vi "SMTP Email [VRFY].vi"(4 "error in (no error)":errorcluster, 6 "user":string, 7 "smtp session":T1) -> (0 "error out":errorcluster, 1 "reply":string, 2 "reply code":i32, 3 "smtp session out":T1)   [LabVIEW 2009, in "NewNI_SMTPEmail.lvlib"]
doc: "Sends the VRFY command to the SMTP server through TCP connection described by \"connection ID\", receives reply and interprets it.\n\nThis VI returns \"connection ID out,\" and the results of the error interpretation to the \"error out\" cluster."
uses:
  NewNI_SMTPEmail.lvlib
  SMTP Email Session.ctl
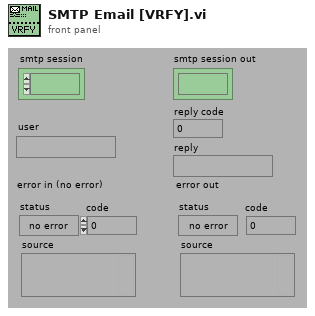
[diagram p1: front panel]
types:
  T1 = typedef "NewNI_SMTPEmail.lvlib/SMTP Email Session.ctl" = refnum<k1>
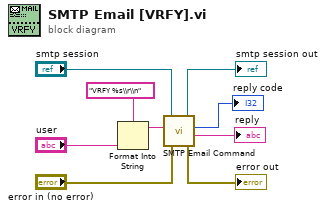
[diagram p0: block diagram]
diagram:
  n1 = Format Into String(format string="VRFY %s\\r\\n", "user") -> (resulting string=w2:string)  [unwired: 2 in, 1 out]
  n2 = call "SMTP Email Command.vi"("error in (no error)"="error in (no error)", "command"=w2, "smtp session"="smtp session") -> ("error out"=→"error out":errorcluster, "reply"=→"reply":string, "reply code"=→"reply code":i32, "smtp session out"=→"smtp session out":T1)  [unwired: 1 out]
